vi "loadEthernetTriggering.vi"(6 "type":string, 8 "error in (no error)":errorcluster, 9 "device.lvclass":refnum<class "device.lvclass">, 10 "xml in":refnum<class "NativeXML.lvclass">, 11 "deviceDataBase in":refnum<class "deviceDataBase.lvclass">) -> (0 "error out":errorcluster, 1 "device.lvclass out":refnum<class "device.lvclass">, 2 "xml out":refnum<class "NativeXML.lvclass">, 3 "deviceDataBase out":refnum<class "deviceDataBase.lvclass">)   [LabVIEW 2009, in "Tools.lvlib" / "DatabaseHelpers.lvlib" / "deviceDataBase.lvclass"]
uses:
  deviceDataBase.lvclass
  Database Objects/device/device.lvclass
  NativeXML/NativeXML.lvclass
  Database Objects/device/EthernetSupply/ethernetSupply.lvclass
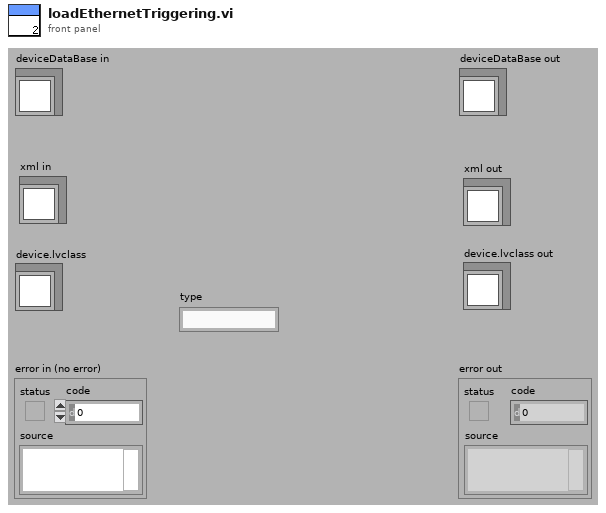
[diagram p1: front panel]
types:
  T1 = cluster{"Range":cluster{"units":string, "min":dbl, "max":dbl}, "triggering_inUse":cluster{"start_trigger":string, "clock":string}, "Limits":cluster{"VoltageLimit":dbl, "CurrentLimit":dbl}}[]
  T2 = cluster{"Range":cluster{"units":string, "min":dbl, "max":dbl}, "triggering_inUse":cluster{"start_trigger":string, "clock":string}, "Limits":cluster{"VoltageLimit":dbl, "CurrentLimit":dbl}}
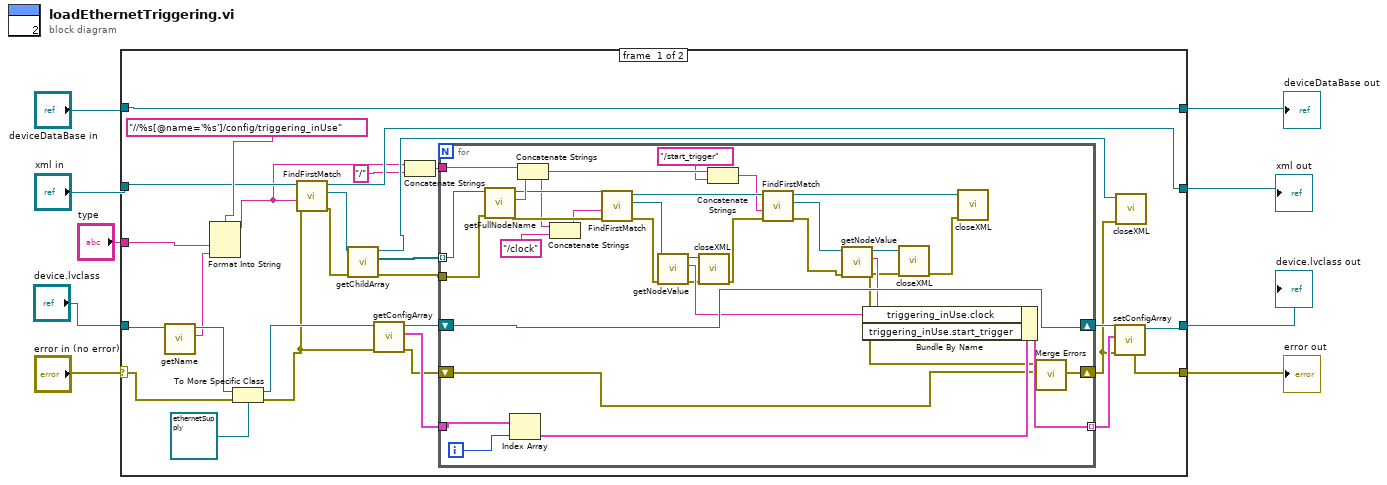
[diagram p0: block diagram]
diagram:
  n1 = case shown="No Error" "error in (no error)" {
    selector: "error in (no error)" -> [w27 w73]
    tunnel: [w28 w73] -> w2
    tunnel: [w37 w72] -> w5
    tunnel: "xml in" -> [w17 w71]
    tunnel: "device.lvclass" -> [w24 w70]
    tunnel: [w29 w70] -> w3
    tunnel: [w16 w71] -> w4
    tunnel: "deviceDataBase in" -> [w37 w72]
    tunnel: "type" -> [w22 _]
    frame #0 {
      n2 = call "getName.vi"("device.lvclass in"=w24) -> ("name"=w21:string, "device.lvclass out"=w23:refnum<class "device.lvclass">)  [unwired: 8 in, 1 out]
      n3 = Format Into String(format string="//%s[@name='%s']/config/triggering_inUse", w22, w21) -> (resulting string=w11:string)  [unwired: 2 in, 1 out]
      n4 = To More Specific Class(target class=refnum<class "ethernetSupply.lvclass"> refnum ("Tools.lvlib:DatabaseHelpers.lvlib:EthernetSupply.lvclass"), reference=w23, error in=w27) -> (specific class reference=w33:refnum<class "ethernetSupply.lvclass">, error out=w15:errorcluster)
      n5 = call "FindFirstMatch.vi"("error in (no error)"=w15, "xPath"=w11, "NativeXML in"=w17) -> ("error out"=w14:errorcluster, "NativeXML match"=w13:refnum<class "NativeXML.lvclass">, "NativeXML out"=w16:refnum<class "NativeXML.lvclass">)  [unwired: 6 in]
      n6 = call "getChildArray.vi"("error in (no error)"=w14, "NativeXML in"=w13) -> ("error out"=w25:errorcluster, "childArray"=w26:refnum<class "NativeXML.lvclass">[], "NativeXML out"=w19:refnum<class "NativeXML.lvclass">)  [unwired: 7 in]
      n7 = call "getConfigArray.vi"("error in (no error)"=w15, "EthernetSupply in"=w33) -> ("error out"=w31:errorcluster, "ConfigArray"=w32:T1, "EthernetSupply out"=w34:refnum<class "ethernetSupply.lvclass">)  [unwired: 7 in]
      n8 = Concatenate Strings(w11, "/") -> (w12:string)
      n9 = for {
        tunnel: w25 -> [w59]
        shift-right: [w64] -> w30
        shift-left: w34 -> [w64]
        shift-right: [w68] -> w18
        shift-left: w31 -> [w63]
        tunnel: w26 -> [w60] mode=indexing
        tunnel: w32 -> [w67]
        tunnel: [w69] -> w35 mode=indexing
        tunnel: w12 -> [w52]
        i -> [w65]
        n10 = call "getFullNodeName.vi"("error in (no error)"=w59, "NativeXML in"=w60) -> ("error out"=w46:errorcluster, "fullName"=w58:string, "NativeXML out"=w50:refnum<class "NativeXML.lvclass">)  [unwired: 7 in]
        n11 = Index Array(array=w67, index=w65) -> (element=w66:T2)
        n12 = Concatenate Strings(w52, w58) -> (w42:string)
        n13 = Concatenate Strings(w42, "/clock") -> (w45:string)
        n14 = call "FindFirstMatch.vi"("error in (no error)"=w46, "xPath"=w45, "NativeXML in"=w50) -> ("error out"=w47:errorcluster, "NativeXML match"=w48:refnum<class "NativeXML.lvclass">, "NativeXML out"=w49:refnum<class "NativeXML.lvclass">)  [unwired: 6 in]
        n15 = call "getNodeValue.vi"("error in (no error)"=w47, "NativeXML in"=w48) -> ("error out"=w56:errorcluster, "Value"=w62:string, "NativeXML out"=w57:refnum<class "NativeXML.lvclass">)  [unwired: 7 in]
        n16 = call "closeXML.vi"("error in (no error)"=w56, "NativeXML in"=w57) -> ("error out"=w44:errorcluster)  [unwired: 9 in]
        n17 = Concatenate Strings(w42, "/start_trigger") -> (w43:string)
        n18 = call "FindFirstMatch.vi"("error in (no error)"=w44, "xPath"=w43, "NativeXML in"=w49) -> ("error out"=w38:errorcluster, "NativeXML match"=w40:refnum<class "NativeXML.lvclass">, "NativeXML out"=w39:refnum<class "NativeXML.lvclass">)  [unwired: 6 in]
        n19 = call "getNodeValue.vi"("error in (no error)"=w38, "NativeXML in"=w40) -> ("error out"=w54:errorcluster, "Value"=w61:string, "NativeXML out"=w55:refnum<class "NativeXML.lvclass">)  [unwired: 7 in]
        n20 = Bundle By Name(cluster=w66, "triggering_inUse.clock"=w62, "triggering_inUse.start_trigger"=w61) -> (w69:T2)
        n21 = call "closeXML.vi"("error in (no error)"=w54, "NativeXML in"=w55) -> ("error out"=w53:errorcluster)  [unwired: 9 in]
        n22 = call "closeXML.vi"("error in (no error)"=w53, "NativeXML in"=w39) -> ()  [unwired: 9 in, 1 out]
        n23 = call <vilib>:"Merge Errors.vi"("error in 2 (no error)"=w63, "error in 1 (no error)"=w54) -> ("error out"=w68:errorcluster)  [unwired: 5 in]
      }
      n24 = call "setConfigArray.vi"("error in (no error)"=w18, "ConfigArray"=w35, "EthernetSupply in"=w30) -> ("error out"=w28:errorcluster, "EthernetSupply out"=w29:refnum<class "ethernetSupply.lvclass">)  [unwired: 7 in]
      n25 = call "closeXML.vi"("error in (no error)"=w18, "NativeXML in"=w19) -> ()  [unwired: 9 in, 1 out]
    }
    frame #1 {
    }
  }
  "error out" <- w2
  "deviceDataBase out" <- w5
  "xml out" <- w4
  "device.lvclass out" <- w3
